vi "PixyCam_Get_Targets.vi"(7 "PixyCamDevRef":T2) -> (1 "ColorCodeTargets Out":T1[](array[typedef]) {"Angle" format="%x"; "Height" format="%x"; "Width" format="%x"; "Y Center" format="%x"; "X Center" format="%x"; "Signature Number" format="%x"; "Checksum" format="%x"; "Target Type" items=["PIXY_START_WORD"=43605, "PIXY_START_WORD_CC"=43606, "PIXY_START_WORDX"=21930]}, 2 "StandardTargets Out":T1[](array[typedef]) {"Angle" format="%x"; "Height" format="%x"; "Width" format="%x"; "Y Center" format="%x"; "X Center" format="%x"; "Signature Number" format="%x"; "Checksum" format="%x"; "Target Type" items=["PIXY_START_WORD"=43605, "PIXY_START_WORD_CC"=43606, "PIXY_START_WORDX"=21930]}, 3 "PixyCamDevRef Out":T2)   [LabVIEW 2016, in "PixyCam_LabVIEW.lvlib"]
uses:
  PixyCam_LabVIEW.lvlib
  Private/PixyCam_DevRef.ctl
  Private/PixyCam_SPI_DevRef.ctl
  <vilib>/Rock Robotics/WPI/SPI/WPI_SPIDevRef.ctl
  <vilib>/Rock Robotics/SystemInterfaces/spilib/spi_bus.ctl
  Private/PixyCam_CommMode.ctl
  Private/PixyCam_TargetData.ctl
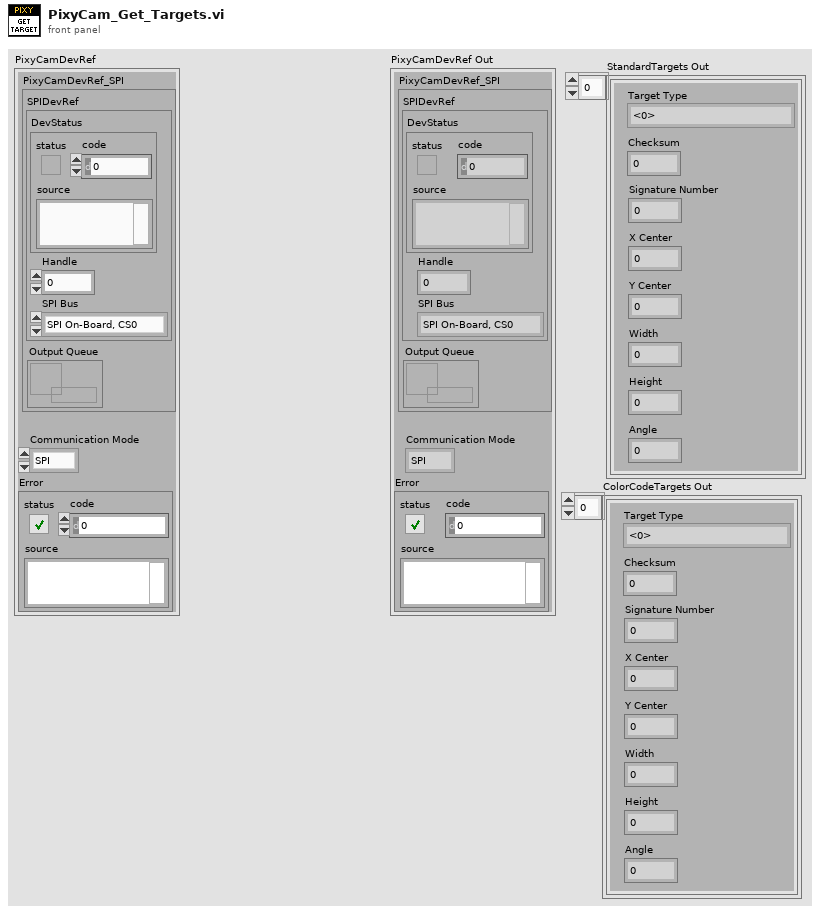
[diagram p1: front panel]
types:
  T1 = typedef "PixyCam_LabVIEW.lvlib/PixyCam_TargetData.ctl" = cluster{"Target Type":u16, "Checksum":u16, "Signature Number":u16, "X Center":u16, "Y Center":u16, "Width":u16, "Height":u16, "Angle":u16}
  T2 = typedef "PixyCam_LabVIEW.lvlib/PixyCam_DevRef.ctl" = cluster{"PixyCamDevRef_SPI":T3, "Communication Mode":T6, "Error":errorcluster}
  T3 = typedef "PixyCam_LabVIEW.lvlib/PixyCam_SPI_DevRef.ctl" = cluster{"SPIDevRef":T4, "Output Queue":refnum<queue>}
  T4 = typedef "WPI_SPIDevRef.ctl" = cluster{"DevStatus":errorcluster, "Handle":i32, "SPI Bus":T5}
  T5 = typedef "spi_bus.ctl" = enum16{"SPI On-Board, CS0", "SPI On-Board, CS1", "SPI On-Board, CS2", "SPI On-Board, CS3", "SPI MXP", "Invalid"}
  T6 = typedef "PixyCam_LabVIEW.lvlib/PixyCam_CommMode.ctl" = enum16{"SPI", "I2C", "UART", "Analog", "Digital"}
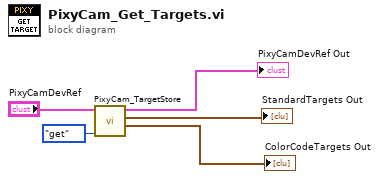
[diagram p0: block diagram]
diagram:
  n1 = call "PixyCam_TargetStore.vi"("Operation"=enum16{"set", "get"}."get", "PixyCamDevRef"="PixyCamDevRef") -> ("ColorCodeTargets Out"=→"ColorCodeTargets Out":T1[], "StandardTargets Out"=→"StandardTargets Out":T1[], "PixyCamDevRef Out"=→"PixyCamDevRef Out":T2)  [unwired: 3 in]
